vi "MAIN - LILI Interface.vi"() -> ()   [LabVIEW 2026]
uses:
  <vilib>/sklein/WebView2/Webview2 Lib/WebView2 Control Object/Paths.ctl
  <vilib>/sklein/WebView2/Webview2 Lib/WebView2 Control Object/Core Env Options.ctl
  <vilib>/sklein/WebView2 QControl/WebView2 QControl/WebView2 QControl/WebView2 QControl.lvclass/WebView2 QControl.ctl
  <userlib>/_lava_lib_tree_control.llb/CommunityTreeAPITYPEDEF - DataStore Command.ctl
  9dcc2fe5-36b0-449a-ab0d-001457c950c8.vi
  5299e24a-5130-419c-9a3c-199b24d92175.vi
  <vilib>/sklein/WebView2 QControl/WebView2 QControl/WebView2 QControl/Write Document Source.vi
  <vilib>/sklein/WebView2 QControl/WebView2 QControl/WebView2 QControl/Read Events.vi
  <vilib>/sklein/WebView2/Webview2 Lib/WebView2 Control Object/Read Events.vi
  <vilib>/sklein/WebView2/Webview2 Lib/WebView2 Control Object/Write Document Source.vi
  <vilib>/sklein/WebView2/Webview2 Lib/WebView2 Control Object/Register Events.vi
  <vilib>/JDP Science/JSONtext/Variant to JSON Text.vi
  <vilib>/JDP Science/JSONtext/LVClass Serializer/JSONtext LVClass Serializer.lvclass
  <vilib>/sklein/WebView2 QControl/WebView2 QControl/WebView2 QControl/WebView2 QControl.lvclass
  <vilib>/sklein/WebView2/Webview2 Lib/WebView2 Control Object/WebView2 Control.lvclass
  <vilib>/sklein/WebView2/Libs/Microsoft.Web.WebView2.WinForms.dll
panel:
  out "<JSON>":string
  in  "WebView2":refnum<k24>(container)
  in  "Bottom Playlist":string(tree)
  in  "Side Playlist":string(tree)
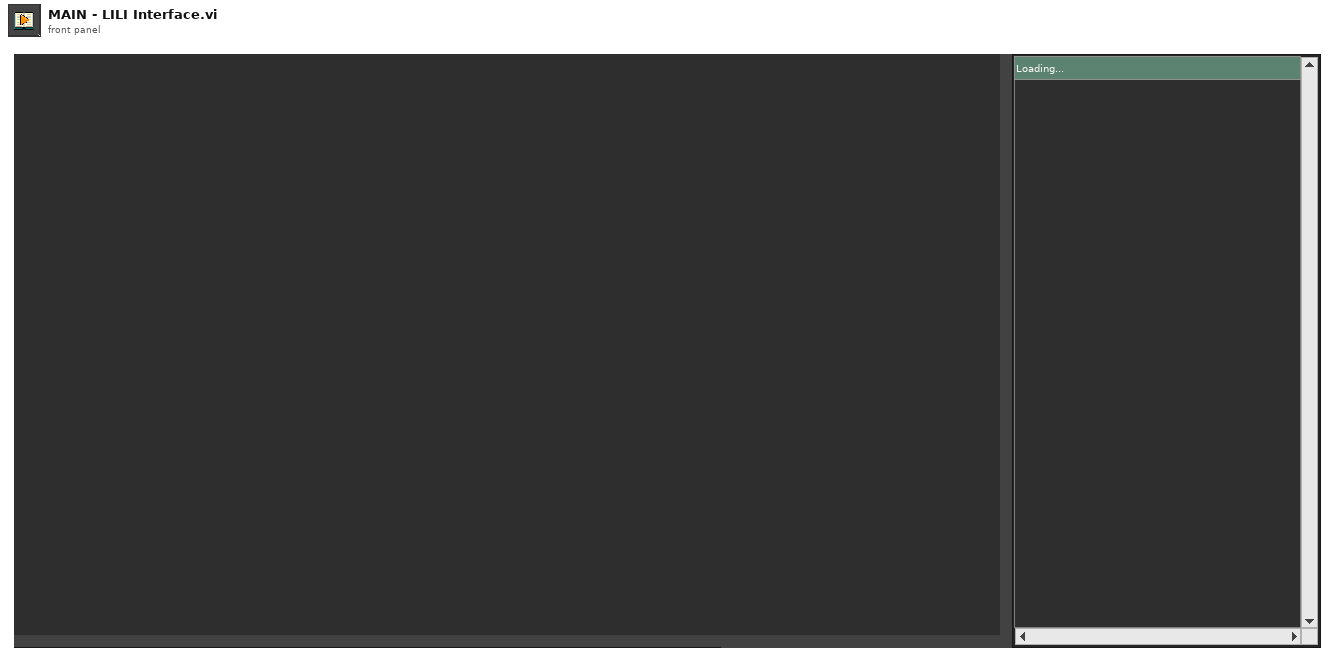
[diagram p1: front panel]
types:
  T1 = typedef "WebView2.lvlib/WebView2 Control.lvclass/Core Env Options.ctl" = cluster{"additionalBrowserArguments":string, "language":string, "targetCompatibleBrowserVersion":string, "allowSingleSignOnUsingOSPrimaryAccount":bool}
  T2 = typedef "WebView2.lvlib/WebView2 Control.lvclass/Paths.ctl" = cluster{"Webview2 Native":path, "Edge Application":path, "User Data":path}
  T3 = typedef "WebView2.lvlib/WebView2 Control.lvclass/Events.ctl" = cluster{"Navigation Complete Event":refnum<user-event>, "Source Changed Event":refnum<user-event>, "Document Title Changed Event":refnum<user-event>, "Status Bar Text Changed":refnum<user-event>, "Web Message Received":refnum<user-event>, "Window Close Requested":refnum<user-event>, "DOM Loaded":refnum<user-event>, "Navigation Started Event":refnum<user-event>}
  T4 = typedef "imagedata.ctl" = cluster{"image type":i32, "image depth":i32, "image":u8[], "mask":u8[], "colors":u32[], "Rectangle":cluster{"left":i16, "top":i16, "right":i16, "bottom":i16}}
  T5 = typedef "CommunityTreeAPITYPEDEF - DataStore Command.ctl" = enum16{"Init", "Add", "Get", "Clear Tree", "Clear All", "Modify"}
  T6 = typedef "LVRectTypeDef.ctl" = cluster{"Left":i16, "Top":i16, "Right":i16, "Bottom":i16}
  T7 = enum16{"No Scaling", "Scale All Objects", "Scale Single Object"}
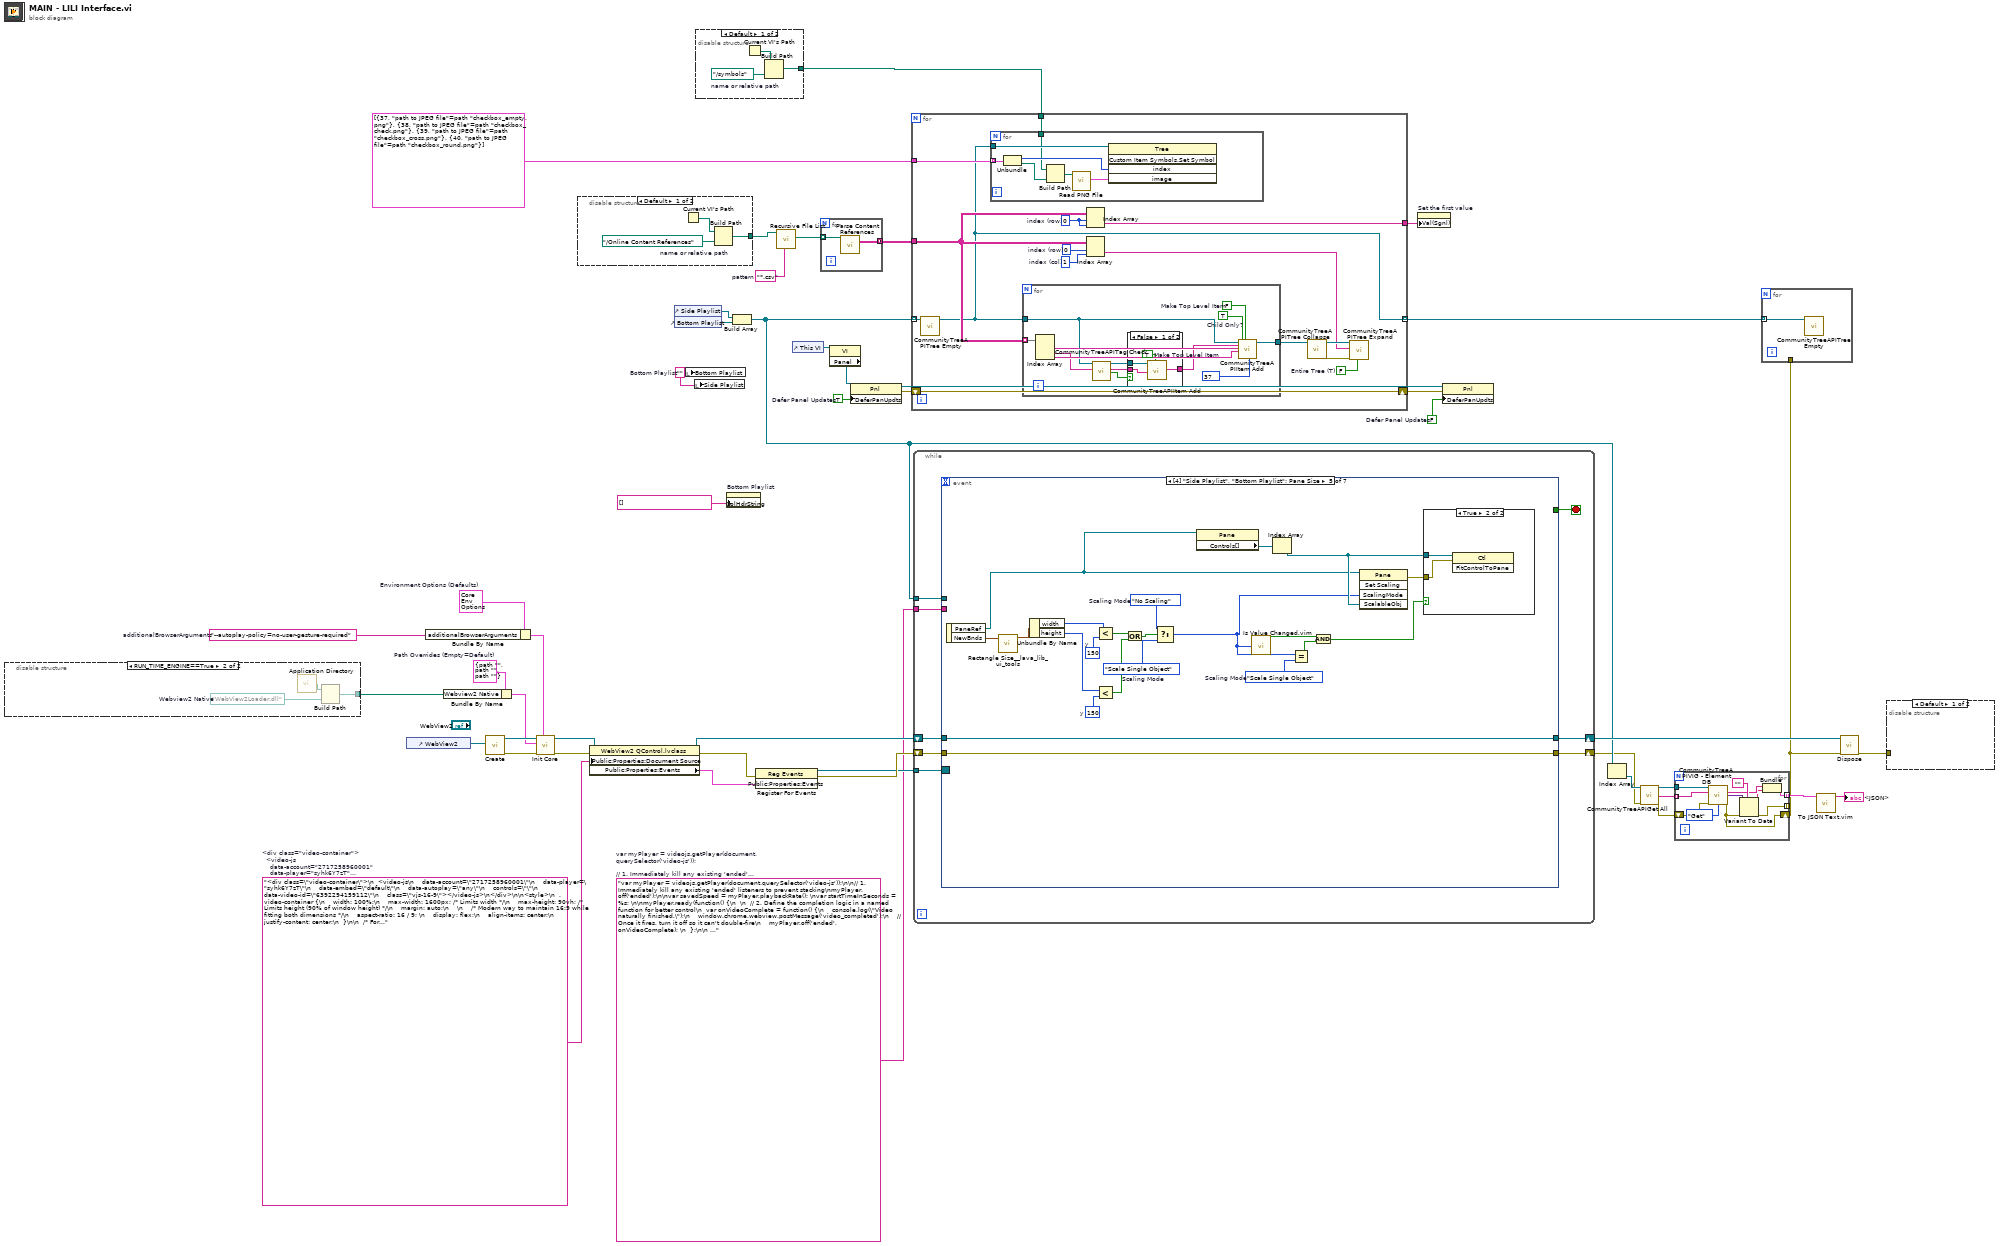
[diagram p0: block diagram]
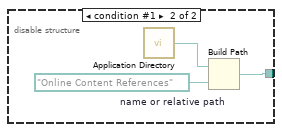
[diagram p2: hidden frame]
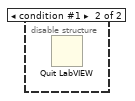
[diagram p4: hidden frame]
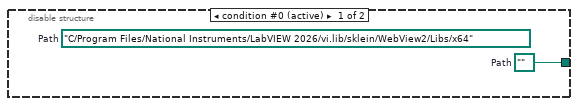
[diagram p5: hidden frame]
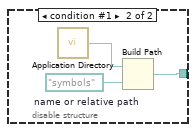
[diagram p6: hidden frame]
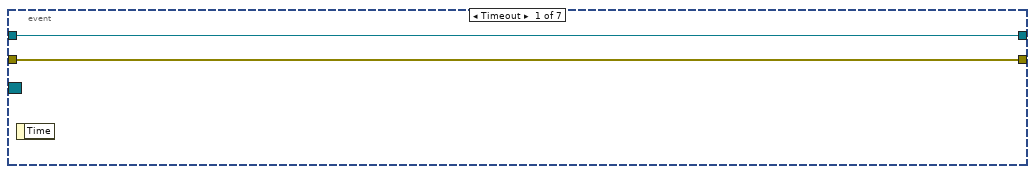
[diagram p7: hidden frame]
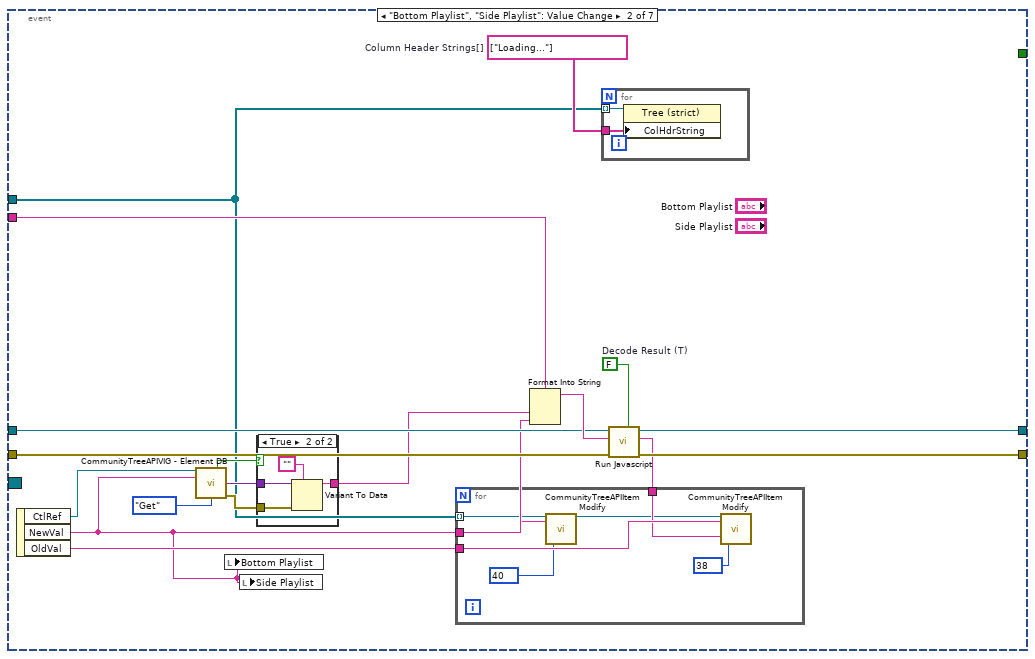
[diagram p8: hidden frame]
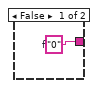
[diagram p9: hidden frame]
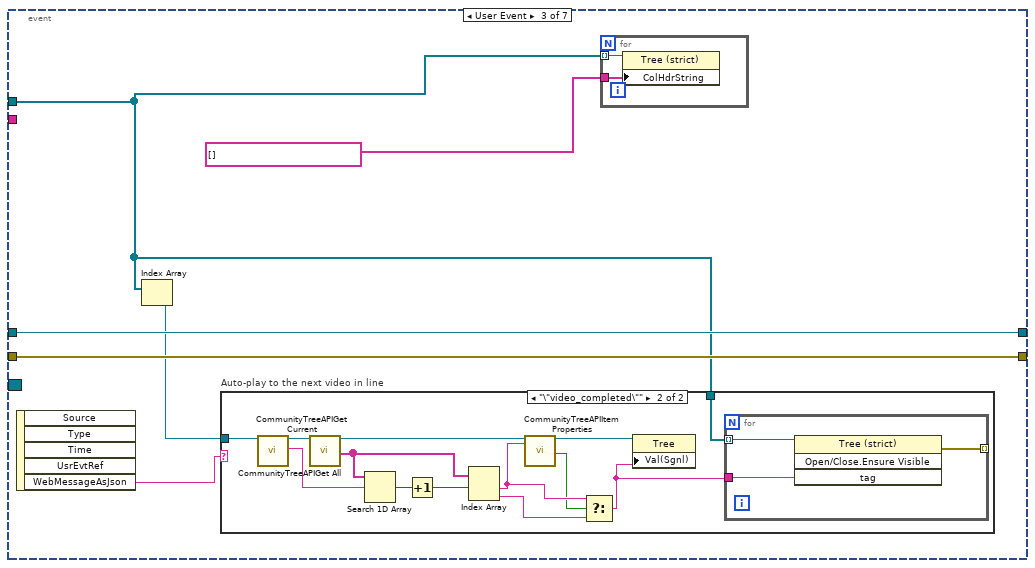
[diagram p10: hidden frame]
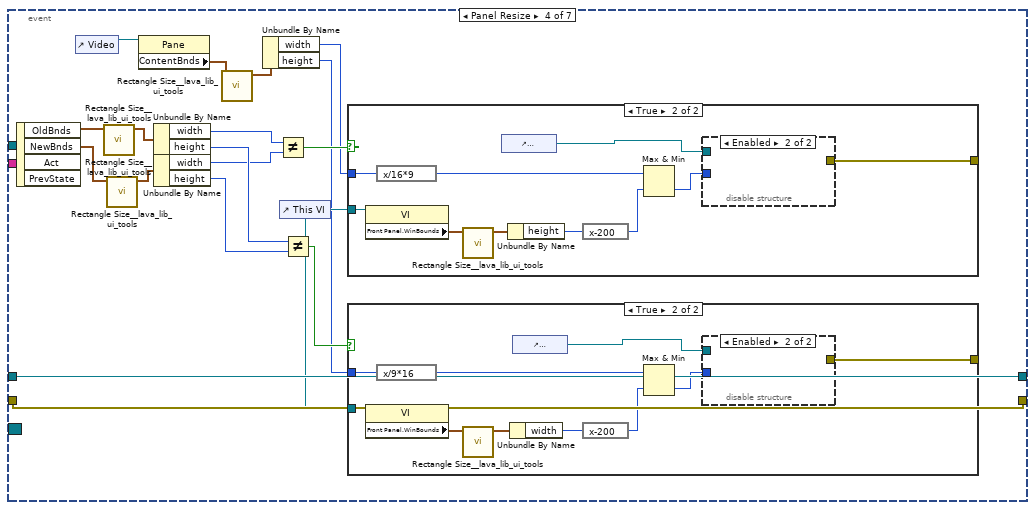
[diagram p12: hidden frame]
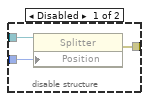
[diagram p14: hidden frame]
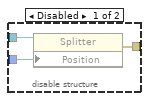
[diagram p16: hidden frame]
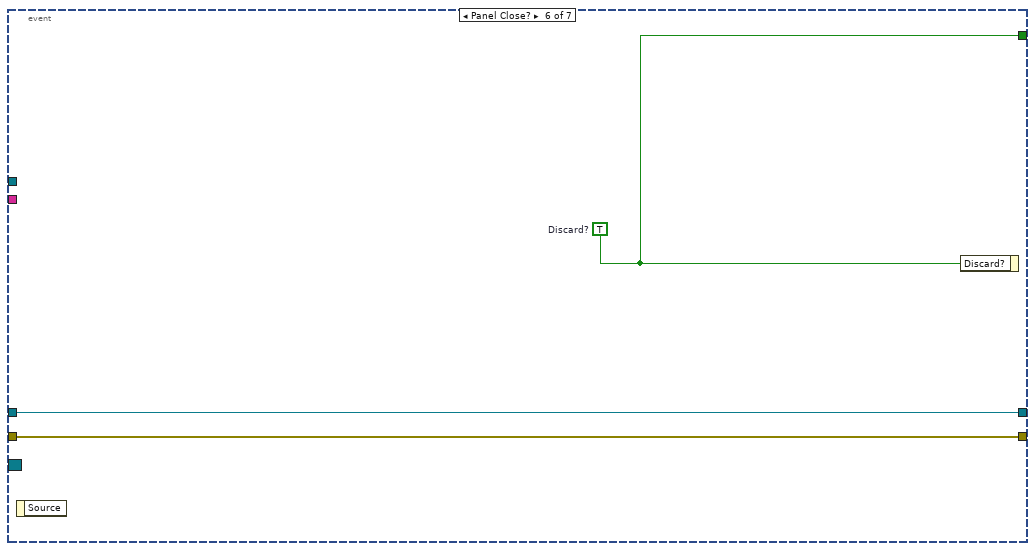
[diagram p18: hidden frame]
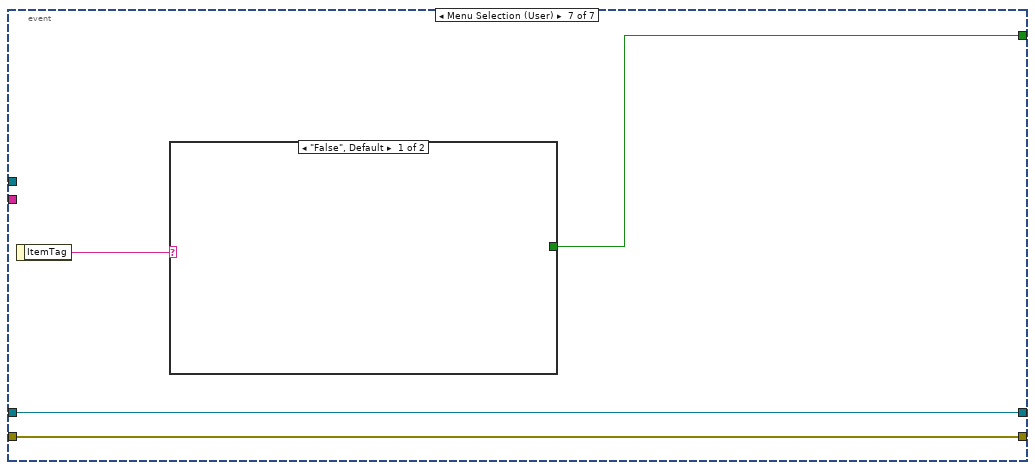
[diagram p19: hidden frame]
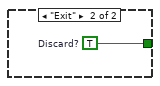
[diagram p20: hidden frame]
diagram:
  w1 = ""  # Bottom Playlist
  w4 = "--autoplay-policy=no-user-gesture-required"  # additionalBrowserArguments
  w6 = T1 {"additionalBrowserArguments"="--autoplay-policy=no-user-gesture-required", "language"="", "targetCompatibleBrowserVersion"="", "allowSingleSignOnUsingOSPrimaryAccount"=FALSE}  # Environment Options (Defaults)
  w18 = "*.csv"  # pattern
  w24 = FALSE  # Defer Panel Updates
  w27 = TRUE  # Defer Panel Updates
  w16 = "var myPlayer = videojs.getPlayer(document.querySelector('video-js'));\n\n// 1. Immediately kill any existing 'ended' listeners to prevent stacking\nmyPlayer.off('ended');\n\nvar savedSpeed = myPlayer.playbackRate(); \nvar startTimeInSeconds = %s; \n\nmyPlayer.ready(function() {\n  \n  // 2. Define the completion logic in a named function for better control\n  var onVideoComplete = function() {\n    console.log(\"Video naturally finished.\");\n    window.chrome.webview.postMessage('video_completed');\n    // Once it fires, turn it off so it can't double-fire\n    myPlayer.off('ended', onVideoComplete); \n  };\n\n  myPlayer.catalog.getVideo('%s', function(error, video) {\n    if (!error) {\n      // 3. Pause and reset the current source before loading the new one\n      myPlayer.pause();\n      \n      myPlayer.catalog.load(video);\n      \n      myPlayer.one('loadedmetadata', function() {\n        myPlayer.playbackRate(savedSpeed);  \n        myPlayer.currentTime(startTimeInSeconds); \n        \n        // 4. Only attach the 'ended' listener AFTER the new video is ready\n        myPlayer.on('ended', onVideoComplete);\n\n        myPlayer.play(); \n        window.chrome.webview.postMessage('abc'); \n      });\n    }\n  });\n});\nmyPlayer.currentTime();"  # var myPlayer = videojs.getPlayer(document.querySelector('video-js'));  // 1. Immediately kill any existing 'ended' listeners to prevent stacking myPlayer.off('ended');  var savedSpeed = myPlayer.playbackRate();  var startTimeInSeconds = %s;   myPlayer.ready(function() {      // 2. Define the completion logic in a named function for better control   var onVideoComplete = function() {     console.log("Video naturally finished.");     window.chrome.webview.postMessage('video_completed');     // Once it fires, turn it off so it can't double-fire     myPlayer.off('ended', onVideoComplete);    };    myPlayer.catalog.getVideo('%s', function(error, video) {     if (!error) {       // 3. Pause and reset the current source before loading the new one       myPlayer.pause();              myPlayer.catalog.load(video);              myPlayer.one('loadedmetadata', function() {         myPlayer.playbackRate(savedSpeed);           myPlayer.currentTime(startTimeInSeconds);                   // 4. Only attach the 'ended' listener AFTER the new video is ready         myPlayer.on('ended', onVideoComplete);          myPlayer.play();          window.chrome.webview.postMessage('abc');        });     }   }); }); myPlayer.currentTime();
  w36 = T2 {"Webview2 Native"=path "", "Edge Application"=path "", "User Data"=path ""}  # Path Overrides (Empty=Default)
  w42 = "<div class=\"video-container\">\n  <video-js\n    data-account=\"2717258960001\"\n    data-player=\"syhk6Y7zT\"\n    data-embed=\"default\"\n    data-autoplay=\"any\"\n    controls=\"\"\n    data-video-id=\"6392294159112\"\n    class=\"vjs-16-9\"></video-js>\n</div>\n\n<style>\n  .video-container {\n    width: 100%;\n    max-width: 1600px; /* Limits width */\n    max-height: 90vh; /* Limits height (90% of window height) */\n    margin: auto;\n    \n    /* Modern way to maintain 16:9 while fitting both dimensions */\n    aspect-ratio: 16 / 9; \n    display: flex;\n    align-items: center;\n    justify-content: center;\n  }\n\n  /* Force the video-js element to fill this constrained container */\n  .video-container video-js {\n    width: 100% !important;\n    height: 100% !important;\n    position: relative !important;\n    padding-top: 0 !important; /* Overrides the default vjs-16-9 padding */\n  }\n</style>\n<script\n  src=\"https://players.brightcove.net/2717258960001/syhk6Y7zT_default/index.min.js\">\n</script>\n"  # <div class="video-container">   <video-js     data-account="2717258960001"     data-player="syhk6Y7zT"     data-embed="default"     data-autoplay="any"     controls=""     data-video-id="6392294159112"     class="vjs-16-9"></video-js> </div>  <style>   .video-container {     width: 100%;     max-width: 1600px; /* Limits width */     max-height: 90vh; /* Limits height (90% of window height) */     margin: auto;          /* Modern way to maintain 16:9 while fitting both dimensions */     aspect-ratio: 16 / 9;      display: flex;     align-items: center;     justify-content: center;   }    /* Force the video-js element to fill this constrained container */   .video-container video-js {     width: 100% !important;     height: 100% !important;     position: relative !important;     padding-top: 0 !important; /* Overrides the default vjs-16-9 padding */   } </style> <script   src="https://players.brightcove.net/2717258960001/syhk6Y7zT_default/index.min.js"> </script>
  n1 = disable-structure shown="RUN_TIME_ENGINE==True" {
    disable-tunnel: [w49 w50] -> w29
    frame condition #0 (active) {
      (unwired) path "C:/Program Files/National Instruments/LabVIEW 2026/vi.lib/sklein/WebView2/Libs/x64"  # Path
      w49 = path ""  # Path
    }
    frame condition #1 {
      w51 = path "WebView2Loader.dll"  # Webview2 Native
      n2 = call <vilib>:"Application Directory.vi"() -> ("Application Directory"=w52:path)
      n3 = Build Path(base path=w52, name or relative path=w51) -> (appended path=w50:path)
    }
  }
  n4 = control-ref of="WebView2"() -> (w46:refnum<vi>)
  n5 = Bundle By Name(cluster=w6, "additionalBrowserArguments"=w4) -> (w5:T1)
  n6 = Bundle By Name(cluster=w36, "Webview2 Native"=w29) -> (w34:T2)
  n7 = call <vilib>:"Create.vi"("WebView2 Control Ref"=w46) -> ("error out"=w40:errorcluster, "WebView2 Control out"=w45:refnum<class "WebView2 QControl.lvclass">)  [unwired: 9 in]
  n8 = call <vilib>:"Init Core.vi"("Environment Options (Defaults)"=w5, "error in (no error)"=w40, "Path Overrides (Empty=Default)"=w34, "WebView2 Control in"=w45) -> ("error out"=w44:errorcluster, "WebView2 Control out"=w39:refnum<class "WebView2 QControl.lvclass">)  [unwired: 6 in]
  n9 = disable-structure shown="Default" {
    disable-tunnel: [w53 w56] -> w19
    frame condition #0 (active) {
      w55 = path "../Online Content References"  # name or relative path
      n10 = Current VI's Path() -> (path=w54:path)
      n11 = Build Path(base path=w54, name or relative path=w55) -> (appended path=w53:path)
    }
    frame condition #1 {
      w58 = path "Online Content References"  # name or relative path
      n12 = call <vilib>:"Application Directory.vi"() -> ("Application Directory"=w57:path)
      n13 = Build Path(base path=w57, name or relative path=w58) -> (appended path=w56:path)
    }
  }
  n14 = property class="WebView2 QControl.lvclass"(reference=w39, error in=w44, "Public:Properties:Document Source"=w42) -> (reference out=w38:refnum<class "WebView2 QControl.lvclass">, error out=w3:errorcluster, "Public:Properties:Events"=w32:T3)
  n15 = control-ref of="Side Playlist"() -> (w28:refnum<vi>)
  n16 = control-ref of="Bottom Playlist"() -> (w47:refnum<vi>)
  n17 = local write "Bottom Playlist"(w1) -> ()
  n18 = local write "Side Playlist"(w1) -> ()
  n19 = disable-structure shown="Default" {
    disable-tunnel: [w59 w62] -> w37
    frame condition #0 (active) {
      w61 = path "../symbols"  # name or relative path
      n20 = Current VI's Path() -> (path=w60:path)
      n21 = Build Path(base path=w60, name or relative path=w61) -> (appended path=w59:path)
    }
    frame condition #1 {
      w64 = path "symbols"  # name or relative path
      n22 = call <vilib>:"Application Directory.vi"() -> ("Application Directory"=w63:path)
      n23 = Build Path(base path=w63, name or relative path=w64) -> (appended path=w62:path)
    }
  }
  n24 = property on="Bottom Playlist" class="Tree (strict)"("ColHdrString"=string[] []) -> ()  [unwired: 2 in, 2 out]
  n25 = Build Array(w28, w47) -> (w15:refnum<vi>[])
  n26 = register-events(error in=w3, w32) -> (reference out=w31:refnum<event-registration>, error out=w48:errorcluster)  [unwired: 1 in]
  n27 = call <vilib>:"Recursive File List.vi"("pattern"=w18, "Folder Path"=w19) -> ("All Files in Dir"=w17:path[])  [unwired: 5 in, 4 out]
  n28 = control-ref of="This VI"() -> (w22:refnum<vi>)
  n29 = for {
    tunnel: [w66] -> w30 mode=concatenating
    tunnel: w17 -> [w65] mode=indexing
    n30 = call "Parse Content References.vi"("file path in"=w65) -> ("transposed array"=w66:string[][])  [unwired: 14 in]
  }
  n31 = property class="VI"(reference=w22) -> ("Panel"=w21:refnum<vi>)  [unwired: 1 in, 2 out]
  n32 = property class="Pnl"(reference=w21, "DeferPanUpdts"=w27) -> (reference out=w23:refnum<vi>, error out=w26:errorcluster)  [unwired: 1 in]
  n33 = for {
    tunnel: w15 -> [w81] mode=indexing
    tunnel: cluster{i32, "path to JPEG file":path}[] [{37, "path to JPEG file"=path "checkbox_empty.png"}, {38, "path to JPEG file"=path "checkbox_check.png"}, {39, "path to JPEG file"=path "checkbox_cross.png"}, {40, "path to JPEG file"=path "checkbox_round.png"}] -> [w80]
    tunnel: w37 -> [w78]
    tunnel: w30 -> [w70]
    shift-right: [w69] -> w25
    shift-left: w26 -> [w69]
    tunnel: [w68] -> w20 mode=indexing
    tunnel: [w67] -> w2
    w72 = 1  # index (col)
    w73 = 0  # index (row)
    w74 = FALSE  # Entire Tree (T)
    w79 = 0  # index (row)
    n34 = call <userlib>:"CommunityTreeAPITree Empty.vi"("Tree Reference In"=w81) -> ("Tree Reference Out"=w68:refnum<vi>)  [unwired: 16 in, 2 out]
    n35 = for {
      tunnel: w68 -> [w88]
      tunnel: w80 -> [w86] mode=indexing
      tunnel: w78 -> [w82]
      n36 = Unbundle(w86) -> (w85:i32, "path to JPEG file"=w84:path)
      n37 = Build Path(base path=w82, name or relative path=w84) -> (appended path=w83:path)
      n38 = call <vilib>:"Read PNG File.vi"("path to PNG file"=w83) -> ("image data"=w87:T4)  [unwired: 8 in, 2 out]
      n39 = invoke class="Tree" method="Custom Item Symbols.Set Symbol"(reference=w88, "index"=w85, "image"=w87) -> ()  [unwired: 2 in, 5 out]
    }
    n40 = for {
      tunnel: w70 -> [w101] mode=indexing
      tunnel: w68 -> [w96]
      tunnel: [w89] -> w77
      w90 = TRUE  # Child Only?
      w98 = FALSE  # Make Top Level Item
      n41 = Index Array(array=w101) -> (element #1=w99:string, element #2=w95:string, element #3=w100:string)  [unwired: 3 in]
      n42 = call <userlib>:"CommunityTreeAPITag Check.vi"("Tree Reference In"=w96, "Input Tag"=w95) -> ("Tree Reference Out"=w94:refnum<vi>, "Duplicate Tag"=w93:string, "Tag OK"=w91:bool)  [unwired: 14 in, 1 out]
      n43 = case shown="False" w91 {
        tunnel: w94 -> [w105 _]
        tunnel: w93 -> [w104 w106]
        tunnel: [w102 w106] -> w92
        frame False {
          w103 = TRUE  # Make Top Level Item
          n44 = call <userlib>:"CommunityTreeAPIItem Add.vi"("Tree Reference In"=w105, "New Text Value"=w104, "Make Top Level Item"=w103) -> ("Created Tag"=w102:string)  [unwired: 14 in, 2 out]
        }
        frame True {
        }
      }
      n45 = call <userlib>:"CommunityTreeAPIItem Add.vi"("Tree Reference In"=w96, "Parent Tag (Current)"=w92, "New Tag Value (Same as Text)"=w99, "New Text Value"=w100, "Child Only?"=w90, "Make Top Level Item"=w98, "Symbol Index (0)"=37) -> ("Tree Reference Out"=w89:refnum<vi>)  [unwired: 10 in, 2 out]
    }
    n46 = Index Array(array=w70, index (row)=w79, index (col)=w79) -> (element=w67:string)
    n47 = Index Array(array=w70, index (row)=w73, index (col)=w72) -> (element=w71:string)
    n48 = call <userlib>:"CommunityTreeAPITree Collapse.vi"("Tree Reference In"=w77) -> ("Tree Reference Out"=w76:refnum<vi>, "error out"=w75:errorcluster)  [unwired: 17 in]
    n49 = call <userlib>:"CommunityTreeAPITree Expand.vi"("Tree Reference In"=w76, "Tag To Expand"=w71, "error in (no error)"=w75, "Entire Tree (T)"=w74) -> ()  [unwired: 14 in, 2 out]
  }
  n50 = while {
    shift-right: [w111] -> w8
    shift-left: w48 -> [w114]
    shift-right: [w112] -> w43
    shift-left: w38 -> [w113]
    tunnel: w31 -> [w109]
    tunnel: w16 -> [w108]
    tunnel: w15 -> [w107]
    stop <- w110 stop-if-true
    n51 = event shown="[4] \"Side Playlist\", \"Bottom Playlist\": Pane Size" {
      selector: w109 -> [_ _ _ _ _ _ _]
      dyn-events: _ -> [_ _ _ _ _ _ _]
      timeout: _ -> [_ _ _ _ _ _ _]
      tunnel: w114 -> [w115 w132 w153 w189 w237 w242 w246]
      tunnel: w113 -> [w116 w130 w154 w190 w238 w243 w247]
      tunnel: [w116 w134 w154 w190 w238 w243 w247] -> w112
      tunnel: [w115 w133 w153 w189 w237 w242 w246] -> w111
      tunnel: [_ _ _ _ _ w241 w244] -> w110
      tunnel: w108 -> [_ w118 _ _ _ _ _]
      tunnel: w107 -> [_ w117 w149 _ _ _ _]
      event Timeout {
        n52 = event-data() -> ()  [unwired: 1 in, 1 out]
      }
      event "Bottom Playlist", "Side Playlist": Value Change {
        w120 = string[] ["Loading..."]  # Column Header Strings[]
        w129 = FALSE  # Decode Result (T)
        n53 = event-data() -> ("CtlRef"=w124:refnum<vi>, "NewVal"=w119:string, "OldVal"=w128:string)  [unwired: 1 in]
        n54 = call <userlib>:"CommunityTreeAPIVIG - Element DB.vi"("Tree Ref In"=w124, "Element Tag"=w119, "Command"=CommunityTreeAPITYPEDEF_-_DataStore_Command."Get") -> ("Found"=w122:bool, "Tree Element Data Out"=w125:variant, "error out"=w123:errorcluster)  [unwired: 7 in, 3 out]
        n55 = local write "Bottom Playlist"(w119) -> ()
        n56 = local write "Side Playlist"(w119) -> ()
        n57 = case shown="True" w122 {
          tunnel: w125 -> [_ w148]
          tunnel: [w144 w146] -> w121
          tunnel: w123 -> [_ w145]
          frame False {
            w144 = "0"  # f
          }
          frame True {
            n58 = Variant To Data(error in=w145, type="", Variant=w148) -> (data=w146:string)  [unwired: 1 out]
          }
        }
        n59 = Format Into String(format string=w118, w121, w119) -> (resulting string=w131:string)  [unwired: 2 in, 1 out]
        n60 = for {
          tunnel: w120 -> [w136]
          tunnel: w117 -> [w135] mode=indexing
          n61 = property on="Property Node" class="Tree (strict)"(reference=w135, "ColHdrString"=w136) -> ()  [unwired: 1 in, 2 out]
        }
        n62 = call <vilib>:"Run Javascript.vi"("Decode Result (T)"=w129, "error in (no error)"=w132, "javaScript"=w131, "WebView2 Control in"=w130) -> ("error out"=w133:errorcluster, "Result"=w127:string, "WebView2 Control out"=w134:refnum<class "WebView2 QControl.lvclass">)  [unwired: 5 in]
        n63 = for {
          tunnel: w128 -> [w143]
          tunnel: w127 -> [w142]
          tunnel: w117 -> [w141] mode=indexing
          tunnel: w119 -> [w137]
          n64 = call <userlib>:"CommunityTreeAPIItem Modify.vi"("Tree Reference In"=w141, "Tag to Modify (Current)"=w137, "Symbol(-1:No Change)"=40) -> ("Tree Reference Out"=w139:refnum<vi>)  [unwired: 14 in, 2 out]
          n65 = call <userlib>:"CommunityTreeAPIItem Modify.vi"("Tree Reference In"=w139, "Tag to Modify (Current)"=w143, "Element Data"=w142, "Symbol(-1:No Change)"=38) -> ()  [unwired: 13 in, 3 out]
        }
      }
      event User Event {
        n66 = event-data() -> ("WebMessageAsJson"=w151:string)  [unwired: 1 in, 4 out]
        n67 = Index Array(array=w149) -> (element=w150:refnum<vi>)  [unwired: 1 in]
        n68 = case "Auto-play to the next video in line" shown="\"\\\"video_completed\\\"\"" w151 {
          tunnel: w150 -> [_ w166]
          tunnel: w149 -> [_ w157]
          frame Default {
          }
          frame "\"video_completed\"" {
            n69 = call <userlib>:"CommunityTreeAPIGet Current.vi"("Tree Reference In"=w166) -> ("Tree Reference Out"=w167:refnum<vi>, "Current Tag"=w165:string)  [unwired: 15 in, 2 out]
            n70 = call <userlib>:"CommunityTreeAPIGet All.vi"("Tree Reference In"=w167) -> ("Tree Reference Out"=w162:refnum<vi>, "Output Tree Items"=w156:string[])  [unwired: 15 in, 2 out]
            n71 = Search 1D Array(1D array=w156, element=w165) -> (index of element=w164:i32)  [unwired: 1 in]
            n72 = Increment(x=w164) -> (x+1=w163:i32)
            n73 = Index Array(array=w156, index #1=w163) -> (element #1=w160:string, element #2=w155:string)  [unwired: 1 in]
            n74 = call <userlib>:"CommunityTreeAPIItem Properties.vi"("Tree Reference In"=w162, "Tag (Current)"=w160) -> ("Tree Reference Out"=w161:refnum<vi>, "Child-Only?"=w159:bool)  [unwired: 10 in, 6 out]
            n75 = Select(t=w160, s=w159, f=w155) -> (s? t:f=w158:string)
            n76 = property on="Property Node" class="Tree"(reference=w161, "Val(Sgnl)"=w158) -> ()  [unwired: 1 in, 2 out]
            n77 = for {
              tunnel: w158 -> [w170]
              tunnel: w157 -> [w169] mode=indexing
              tunnel: [w168] -> _ mode=indexing
              n78 = invoke class="Tree (strict)" method="Open/Close.Ensure Visible"(reference=w169, "tag"=w170) -> (error out=w168:errorcluster)  [unwired: 2 in, 3 out]
            }
          }
        }
        n79 = for {
          tunnel: string[] [] -> [w172]
          tunnel: w149 -> [w171] mode=indexing
          n80 = property on="Property Node" class="Tree (strict)"(reference=w171, "ColHdrString"=w172) -> ()  [unwired: 1 in, 2 out]
        }
      }
      event Panel Resize {
        n81 = event-data() -> ("OldBnds"=w188:T6, "NewBnds"=w183:T6)  [unwired: 1 in, 2 out]
        n82 = control-ref of="Video"() -> (w179:refnum<vi>)
        n83 = call <vilib>:"Rectangle Size__lava_lib_ui_tools.vi"("Rectangle"=w188) -> ("Rect Size"=w187:cluster{"width":i32, "height":i32})  [unwired: 8 in, 2 out]
        n84 = call <vilib>:"Rectangle Size__lava_lib_ui_tools.vi"() -> ()  [unwired: 9 in, 3 out]
        n85 = call <vilib>:"Rectangle Size__lava_lib_ui_tools.vi"("Rectangle"=w183) -> ("Rect Size"=w186:cluster{"width":i32, "height":i32})  [unwired: 8 in, 2 out]
        n86 = property class="Pane"(reference=w179) -> ("ContentBnds"=w178:T6)  [unwired: 1 in, 2 out]
        n87 = Unbundle By Name(w187) -> ("width"=w185:i32, "height"=w182:i32)
        n88 = Unbundle By Name(w186) -> ("width"=w176:i32, "height"=w174:i32)
        n89 = call <vilib>:"Rectangle Size__lava_lib_ui_tools.vi"("Rectangle"=w178) -> ("Rect Size"=w177:cluster{"width":i32, "height":i32})  [unwired: 8 in, 2 out]
        n90 = Unbundle By Name(w177) -> ("width"=w175:i32, "height"=w173:i32)
        n91 = Not Equal?(x=w185, y=w176) -> (x != y?=w184:bool)
        n92 = control-ref of="This VI"() -> (w180:refnum<vi>)
        n93 = Not Equal?(x=w182, y=w174) -> (x != y?=w181:bool)
        n94 = case shown="True" w184 {
          tunnel: w175 -> [_ w213]
          tunnel: [_ w211] -> _
          tunnel: w180 -> [_ w209]
          frame False {
          }
          frame True {
            n95 = property class="VI"(reference=w209) -> ("Front Panel.WinBounds"=w208:T6)  [unwired: 1 in, 2 out]
            n96 = expression code="x/16*9"(w213) -> (w212:i32)
            n97 = call <vilib>:"Rectangle Size__lava_lib_ui_tools.vi"("Rectangle"=w208) -> ("Rect Size"=w207:cluster{"width":i32, "height":i32})  [unwired: 8 in, 2 out]
            n98 = control-ref of="Video<>Bottom"() -> (w204:refnum<vi>)
            n99 = Unbundle By Name(w207) -> ("height"=w206:i32)
            n100 = expression code="x-200"(w206) -> (w205:i32)
            n101 = Max & Min(x=w212, y=w205) -> (min(x,y)=w210:i32)  [unwired: 1 out]
            n102 = disable-structure shown="Enabled" {
              disable-tunnel: w204 -> [w216 _]
              disable-tunnel: [w215 _] -> w211
              disable-tunnel: w210 -> [w214 _]
              frame Disabled {
                n103 = property class="Splitter"(reference=w216, "Position"=w214) -> (error out=w215:errorcluster)  [unwired: 1 in, 1 out]
              }
              frame Enabled {
              }
            }
          }
        }
        n104 = case shown="True" w181 {
          tunnel: [_ w199] -> _
          tunnel: w180 -> [_ w197]
          tunnel: w173 -> [_ w192]
          frame False {
          }
          frame True {
            n105 = property class="VI"(reference=w197) -> ("Front Panel.WinBounds"=w196:T6)  [unwired: 1 in, 2 out]
            n106 = expression code="x/9*16"(w192) -> (w200:i32)
            n107 = call <vilib>:"Rectangle Size__lava_lib_ui_tools.vi"("Rectangle"=w196) -> ("Rect Size"=w195:cluster{"width":i32, "height":i32})  [unwired: 8 in, 2 out]
            n108 = Unbundle By Name(w195) -> ("width"=w194:i32)
            n109 = control-ref of="Video<>Side"() -> (w191:refnum<vi>)
            n110 = expression code="x-200"(w194) -> (w193:i32)
            n111 = Max & Min(x=w200, y=w193) -> (min(x,y)=w198:i32)  [unwired: 1 out]
            n112 = disable-structure shown="Enabled" {
              disable-tunnel: w191 -> [w203 _]
              disable-tunnel: [w202 _] -> w199
              disable-tunnel: w198 -> [w201 _]
              frame Disabled {
                n113 = property class="Splitter"(reference=w203, "Position"=w201) -> (error out=w202:errorcluster)  [unwired: 1 in, 1 out]
              }
              frame Enabled {
              }
            }
          }
        }
      }
      event Pane Size {
        w220 = 150  # y
        w225 = T7."Scale Single Object"  # Scaling Mode
        w231 = T7."Scale Single Object"  # Scaling Mode
        w230 = T7."No Scaling"  # Scaling Mode
        w233 = 150  # y
        n114 = event-data() -> ("PaneRef"=w221:refnum<vi>, "NewBnds"=w236:T6)  [unwired: 1 in]
        n115 = call <vilib>:"Rectangle Size__lava_lib_ui_tools.vi"("Rectangle"=w236) -> ("Rect Size"=w235:cluster{"width":i32, "height":i32})  [unwired: 8 in, 2 out]
        n116 = Unbundle By Name(w235) -> ("width"=w234:i32, "height"=w219:i32)
        n117 = Less?(x=w234, y=w233) -> (x < y?=w232:bool)
        n118 = Less?(x=w219, y=w220) -> (x < y?=w217:bool)
        n119 = Or(x=w232, y=w217) -> (x .or. y?=w218:bool)
        n120 = Select(t=w230, s=w218, f=w231) -> (s? t:f=w224:T7)
        n121 = property class="Pane"(reference=w221) -> ("Controls[]"=w229:refnum<vi>[])  [unwired: 1 in, 2 out]
        n122 = call "Is Value Changed.vim"("value"=w224) -> ("changed or first call?"=w226:bool)
        n123 = Index Array(array=w229) -> (element=w228:refnum<vi>)  [unwired: 1 in]
        n124 = Equal?(x=w224, y=w225) -> (x = y?=w223:bool)
        n125 = And(x=w226, y=w223) -> (x .and. y?=w222:bool)
        n126 = invoke class="Pane" method="Set Scaling"(reference=w221, "ScalingMode"=w224, "ScalableObj"=w228) -> (error out=w227:errorcluster)  [unwired: 2 in, 4 out]
        n127 = case shown="True" w222 {
          tunnel: w228 -> [_ w240]
          tunnel: w227 -> [_ w239]
          frame False {
          }
          frame True {
            n128 = invoke class="Ctl" method="FitControlToPane"(reference=w240, error in=w239) -> ()  [unwired: 1 in, 3 out]
          }
        }
      }
      event Panel Close? {
        w241 = TRUE  # Discard?
        n129 = event-data() -> ()  [unwired: 1 in, 1 out]
        n130 = event-data("Discard?"=w241) -> ()  [unwired: 1 in, 1 out]
      }
      event Menu Selection (User) {
        n131 = event-data() -> ("ItemTag"=w245:string)  [unwired: 1 in]
        n132 = case shown="\"False\", Default" w245 {
          tunnel: [_ w248] -> w244
          frame "False", Default {
          }
          frame "Exit" {
            w248 = TRUE  # Discard?
          }
        }
      }
    }
  }
  n133 = property on="Set the first value" class="Tree (strict)"("Val(Sgnl)"=w2) -> ()  [unwired: 2 in, 2 out]
  n134 = property class="Pnl"(reference=w23, error in=w25, "DeferPanUpdts"=w24) -> ()  [unwired: 2 out]
  n135 = Index Array(array=w15) -> (element=w14:refnum<vi>)  [unwired: 1 in]
  n136 = call <userlib>:"CommunityTreeAPIGet All.vi"("Tree Reference In"=w14, "error in (no error)"=w8) -> ("Tree Reference Out"=w13:refnum<vi>, "Output Tree Items"=w12:string[], "error out"=w9:errorcluster)  [unwired: 14 in, 1 out]
  n137 = for {
    tunnel: w13 -> [w258]
    tunnel: w12 -> [w257] mode=indexing
    tunnel: [w252] -> w11 mode=indexing
    shift-right: [w250] -> w7
    shift-left: w9 -> [w251]
    tunnel: [w249] -> _ mode=indexing
    n138 = call <userlib>:"CommunityTreeAPIVIG - Element DB.vi"("Tree Ref In"=w258, "Element Tag"=w257, "error in (no error)"=w251, "Command"=CommunityTreeAPITYPEDEF_-_DataStore_Command."Get") -> ("Element Tag Out"=w254:string, "Tree Element Data Out"=w256:variant, "error out"=w250:errorcluster)  [unwired: 6 in, 3 out]
    n139 = Variant To Data(error in=w250, type="", Variant=w256) -> (data=w253:string, error out=w249:errorcluster)
    n140 = Bundle("Element Tag Out"=w254, w253) -> (w252:cluster{"Element Tag Out":string, string})  [unwired: 1 in]
  }
  n141 = for {
    tunnel: w20 -> [w260] mode=indexing
    tunnel: w7 -> [_]
    n142 = call <userlib>:"CommunityTreeAPITree Empty.vi"("Tree Reference In"=w260) -> ()  [unwired: 16 in, 3 out]
  }
  n143 = call "To JSON Text.vim"("Anything"=w11) -> ("<JSON>"=→"<JSON>":string)  [unwired: 9 in, 1 out]
  n144 = call <vilib>:"Dispose.vi"("error in (no error)"=w7, "WebView2 Control in"=w43) -> ("error out"=w35:errorcluster)  [unwired: 9 in]
  n145 = disable-structure shown="Default" {
    disable-tunnel: w35 -> [_ _]
    frame condition #0 (active) {
    }
    frame condition #1 {
      n146 = Quit LabVIEW() -> ()  [unwired: 1 in]
    }
  }
